vi "Fetch VI Methods Info.vi"(5 "Parser Settings":T9, 8 "Error in":errorcluster caption="Error in (no error)", 9 "Fetch Controls?":bool, 11 "VI Reference":refnum<vi>) -> (0 "Error out":errorcluster, 2 "VI Info":T1)   [LabVIEW 2023, in "VIDoc Parsing.lvlib"]
uses:
  VIDoc Parsing.lvlib
  TypeDefs/VI Type Extended Enum.ctl
  TypeDefs/Class Dispatch Type Enum.ctl
  <vilib>/picture/picture.llb/imagedata.ctl
  <vilib>/Utility/miscctls.llb/LVKeyTypeDef.ctl
  TypeDefs/Controls Info Cluster.ctl
  <vilib>/Utility/miscctls.llb/LVPointTypeDef.ctl
  TypeDefs/Method Spec Cluster.ctl
  Settings/Parser Settings/Draw Option Enum.ctl
  Settings/Parser Settings/Parser Settings.lvclass
  Settings/Parser Settings/Draw Controls Cluster.ctl
  Settings/Parser Settings/Parser Settings Cluster.ctl
  Structure Reporter/Tree Cluster.ctl
  Structure Reporter/Structure Reporter.lvlib
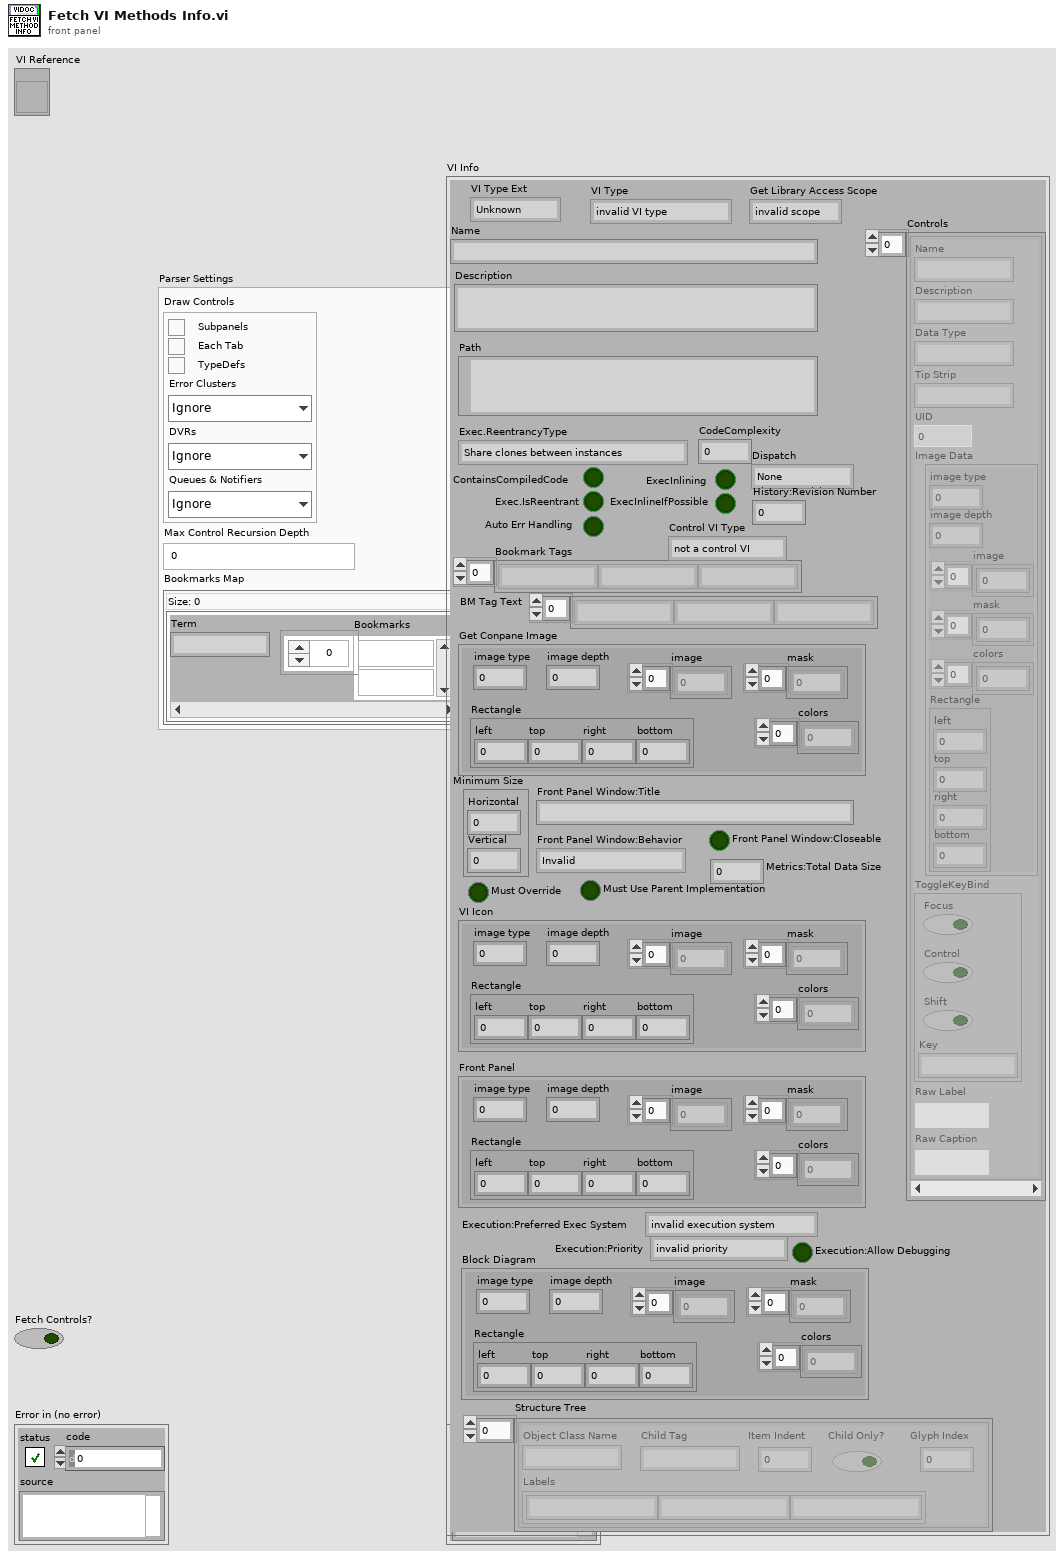
[diagram p1: front panel]
types:
  T1 = typedef "VIDoc Parsing.lvlib/Method Spec Cluster.ctl" = cluster{"VI Type Ext":T2, "Name":string, "Path":path, "Get Conpane Image":T3, "Description":string, "Get Library Access Scope":enum32{"invalid scope", "public", "private", "protected", "community"}, "Dispatch":T4, "ContainsCompiledCode":bool, "Exec.IsReentrant":bool, "Exec.ReentrancyType":enum16{"Share clones between instances", "Preallocate clone for each instance"}, "ExecInlining":bool, "ExecInlineIfPossible":bool, "Auto Err Handling":bool, "CodeComplexity":sgl, "Bookmark Tags":string[], "Control VI Type":enum32{"not a control VI", "control", "typedef", "strict typedef"}, "Controls":T5[], "VI Type":enum32{"invalid VI type", "Standard VI", "Control VI", "Global VI", "Polymorphic VI", "Configuration VI", "SubSystem", "Facade VI", "Method VI", "Statechart Diagram VI"}, "Minimum Size":T7, "Front Panel Window:Title":string, "Front Panel Window:Behavior":enum32{"Invalid", "Default", "Floating", "Floating/Auto-Hide", "Modal"}, "Front Panel Window:Closeable":bool, "Must Override":bool, "Must Use Parent Implementation":bool, "VI Icon":T3, "Front Panel":T3, "History:Revision Number":u32, "Metrics:Total Data Size":u32, "Execution:Allow Debugging":bool, "Execution:Preferred Exec System":enum32{"invalid execution system", "user interface", "standard", "instrument i/o", "data acquisition", "other 1", "other 2", "same as caller"}, "Execution:Priority":enum32{"invalid priority", "background priority", "normal priority", "above normal priority", "high priority", "time critical priority", "subroutine"}, "BM Tag Text":string[], "Block Diagram":T3, "Structure Tree":T8[]}
  T2 = typedef "VIDoc Parsing.lvlib/VI Type Extended Enum.ctl" = enum16{"Unknown", "Class Method", "Class Accessor Get", "Class Accessor Set", "Class Control", "Library Method", "Library Control", "VI", "Control"}
  T3 = typedef "imagedata.ctl" = cluster{"image type":i32, "image depth":i32, "image":u8[], "mask":u8[], "colors":u32[], "Rectangle":cluster{"left":i16, "top":i16, "right":i16, "bottom":i16}}
  T4 = typedef "VIDoc Parsing.lvlib/Class Dispatch Type Enum.ctl" = enum16{"None", "Static", "Dynamic"}
  T5 = typedef "VIDoc Parsing.lvlib/Controls Info Cluster.ctl" = cluster{"Name":string, "Description":string, "Data Type":string, "Tip Strip":string, "UID":i32, "Image Data":T3, "ToggleKeyBind":T6, "Raw Label":string, "Raw Caption":string}
  T6 = typedef "LVKeyTypeDef.ctl" = cluster{"Focus":bool, "Control":bool, "Shift":bool, "Key":string}
  T7 = typedef "LVPointTypeDef.ctl" = cluster{"Horizontal":i16, "Vertical":i16}
  T8 = typedef "VIDoc Parsing.lvlib/Structure Reporter.lvlib/Tree Cluster.ctl" = cluster{"Object Class Name":string, "Labels":string[], "Child Tag":string, "Item Indent":i32, "Child Only?":bool, "Glyph Index":i32}
  T9 = typedef "VIDoc Parsing.lvlib/Parser Settings.lvclass/Parser Settings Cluster.ctl" = cluster{"Draw Controls":T10, "Max Control Recursion Depth":i32, "Bookmarks Map":map{string, string[]}}
  T10 = typedef "VIDoc Parsing.lvlib/Parser Settings.lvclass/Draw Controls Cluster.ctl" = cluster{"Subpanels":bool, "Tabs":bool, "TypeDefs":bool, "Error Clusters":T11, "DVRs":T11, "Queues & Notifiers":T11}
  T11 = typedef "VIDoc Parsing.lvlib/Parser Settings.lvclass/Draw Option Enum.ctl" = enum16{"Ignore", "Draw", "Draw + Contents"}
  T12 = enum32{"invalid VI type", "Standard VI", "Control VI", "Global VI", "Polymorphic VI", "Configuration VI", "SubSystem", "Facade VI", "Method VI", "Statechart Diagram VI"}
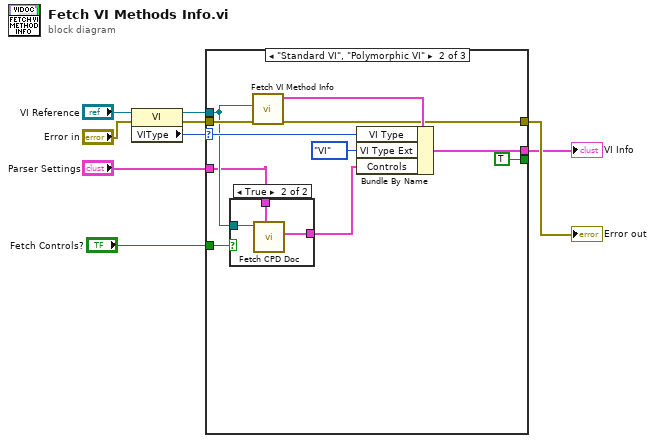
[diagram p0: block diagram]
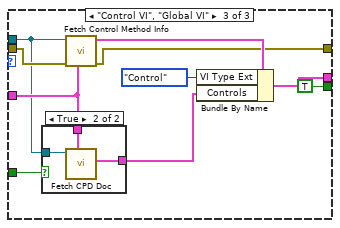
[diagram p4: hidden frame]
diagram:
  n1 = property class="VI"(reference="VI Reference", error in="Error in") -> (reference out=w6:refnum<vi>, error out=w5:errorcluster, "VIType"=w7:T12)
  n2 = case shown="\"Standard VI\", \"Polymorphic VI\"" w7 {
    selector: w7 -> [_ w20 _]
    tunnel: w6 -> [_ w14 w26]
    tunnel: [_ w19 w33] -> w2
    tunnel: [_ TRUE TRUE] -> _
    tunnel: w5 -> [w10 w17 w31]
    tunnel: [w10 w16 w30] -> w9
    tunnel: "Parser Settings" -> [_ w13 w27]
    tunnel: "Fetch Controls?" -> [_ w11 w28]
    frame Default {
    }
    frame "Standard VI", "Polymorphic VI" {
      n3 = case shown="True" w11 {
        tunnel: w14 -> [_ w24]
        tunnel: w13 -> [_ w23]
        tunnel: [_ w22] -> w12
        frame False {
        }
        frame True {
          n4 = call "Fetch CPD Doc.vi"("Parser Settings"=w23, "VI in"=w24) -> ("Class Private Data"=w22:T5[])  [unwired: 8 in, 1 out]
        }
      }
      n5 = call "Fetch VI Method Info.vi"("Error in"=w17, "VI Reference"=w14) -> ("Error out"=w16:errorcluster, "Method Spec Cluster"=w18:T1)  [unwired: 8 in]
      n6 = Bundle By Name(cluster=w18, "VI Type"=w20, "VI Type Ext"=VI_Type_Extended_Enum."VI", "Controls"=w12) -> (w19:T1)
    }
    frame "Control VI", "Global VI" {
      n7 = case shown="True" w28 {
        tunnel: w26 -> [_ w37]
        tunnel: w27 -> [_ w36]
        tunnel: [_ w35] -> w25
        frame False {
        }
        frame True {
          n8 = call "Fetch CPD Doc.vi"("Parser Settings"=w36, "VI in"=w37) -> ("Class Private Data"=w35:T5[])  [unwired: 8 in, 1 out]
        }
      }
      n9 = call "Fetch Control Method Info.vi"("Parser Settings"=w27, "Error in"=w31, "VI in"=w26) -> ("Error out"=w30:errorcluster, "Method Spec Cluster"=w32:T1)  [unwired: 7 in]
      n10 = Bundle By Name(cluster=w32, "VI Type Ext"=VI_Type_Extended_Enum."Control", "Controls"=w25) -> (w33:T1)
    }
  }
  "Error out" <- w9
  "VI Info" <- w2
